vi "plot_point.vi"(8 "Error In":errorcluster) -> (0 "Error Out":errorcluster)   [LabVIEW 2012]
doc: "Given a 3x3 homogenous transformation (T) this function outputs a cluster of the plot components (TrPlot) needed to represent the transformation on an XY Graph."
panel:
  in  "Point Array":dbl[][](array[numeric])
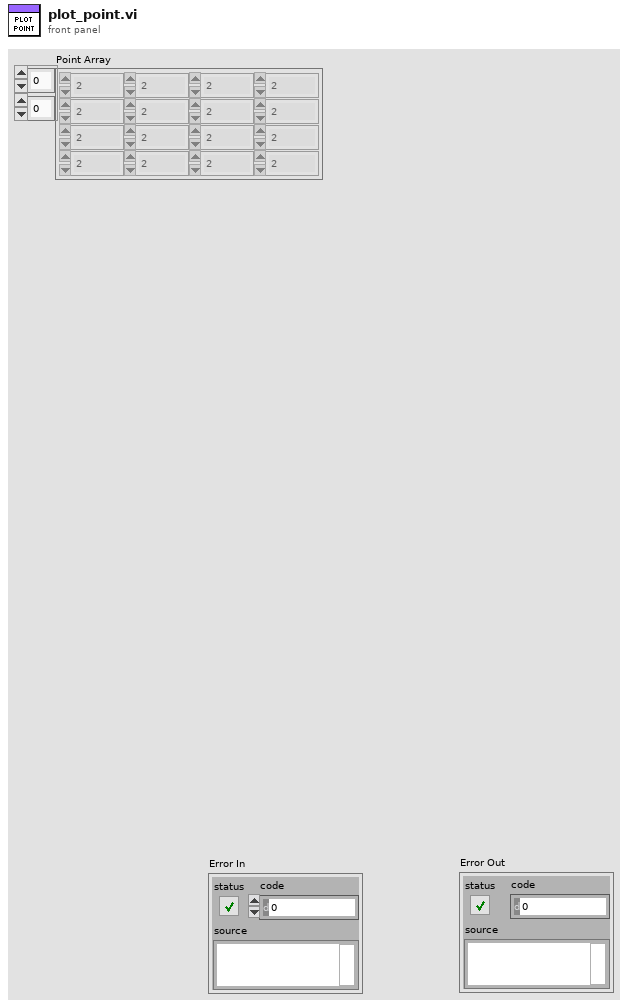
[diagram p1: front panel]
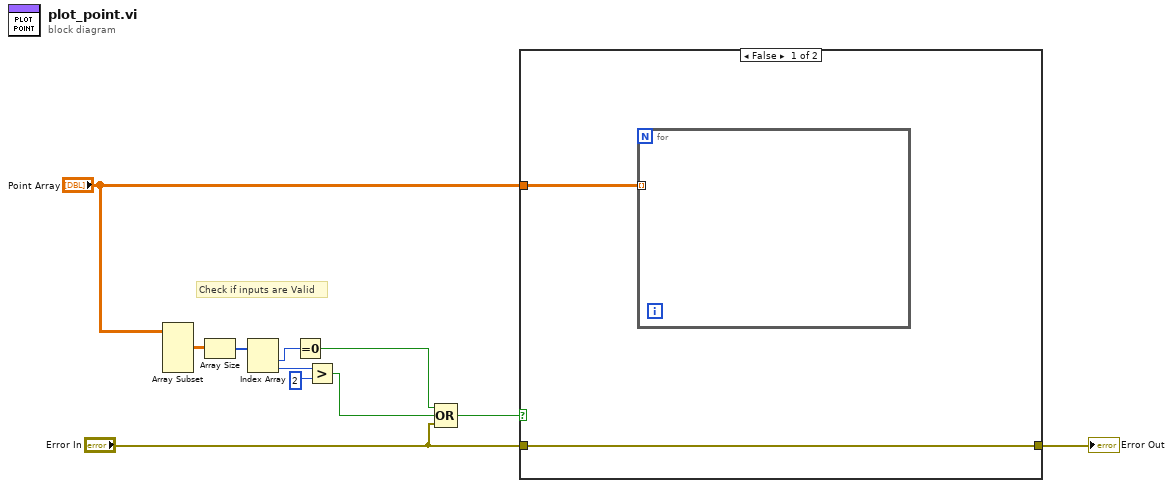
[diagram p0: block diagram]
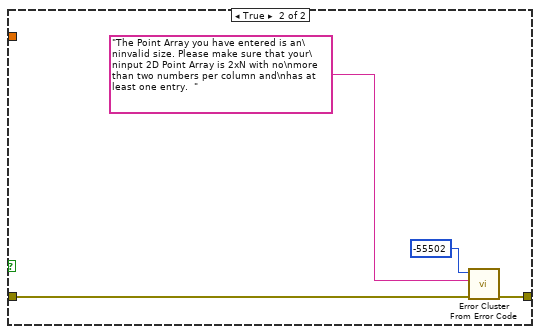
[diagram p2: hidden frame]
diagram:
  # "Check if inputs are Valid"
  n1 = Array Subset(array="Point Array") -> (w11:dbl[][])  [unwired: 4 in]
  n2 = Array Size(array=w11) -> (size(s)=w8:i32[])
  n3 = Index Array(array=w8) -> (element #1=w7:i32, element #2=w6:i32)  [unwired: 2 in]
  n4 = Equal To 0?(x=w7) -> (x = 0?=w5:bool)
  n5 = Greater?(x=w6, y=2) -> (0:w4:bool)
  n6 = Compound Arithmetic op=OR(w5, w4, "Error In") -> (w3:bool)
  n7 = case shown="False" w3 {
    tunnel: "Point Array" -> [w13 _]
    tunnel: [w12 w15] -> w1
    tunnel: "Error In" -> [w12 w16]
    frame False {
      n8 = for {
        tunnel: w13 -> [_] mode=indexing
      }
    }
    frame True {
      n9 = call <vilib>:"Error Cluster From Error Code.vi"("error in (no error)"=w16, "error message (\"\")"="The Point Array you have entered is an\ninvalid size. Please make sure that your\ninput 2D Point Array is 2xN with no\nmore than two numbers per column and\nhas at least one entry.  " ("error message (\"\")"), "error code (0)"=-55502) -> ("error out"=w15:errorcluster)  [unwired: 6 in]
    }
  }
  "Error Out" <- w1
